vi "Combine Vectors.vi"(10 "Rotation Module Data":T1 {"Angle" scale format="%.3f"; "Velocity" scale=-1.0..1.0 scale format="%.1f"}, 11 "Travers Module Data":T1 {"Angle" scale format="%.3f"; "Velocity" scale=-1.0..1.0 scale format="%.1f"}) -> (2 "Velocity Out":dbl, 3 "Combine Out":T1 {"Angle" scale format="%.3f"; "Velocity" scale=-1.0..1.0 scale format="%.1f"})   [LabVIEW 2023, in "SwerveDrive_ACT.lvlib"]
uses:
  SwerveDrive_ACT.lvlib
  Shared Code/TypeDefs/Cluster_Module Velocity-Direction-Rotations.ctl
  Shared Code/TypeDefs/Level_Velocity plus-minus 1.ctl
  Shared Code/TypeDefs/Dial_Compase heading unit circle CCW positive.ctl
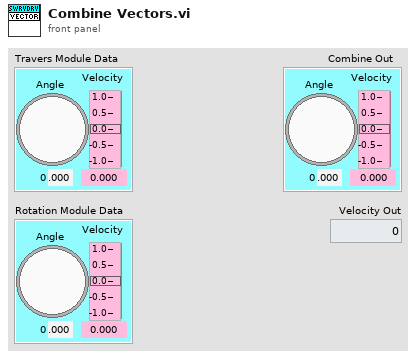
[diagram p1: front panel]
types:
  T1 = typedef "Cluster_Module Velocity-Direction-Rotations.ctl" = cluster{"Velocity":T2, "Angle":T3, "Rotations Count":dbl}
  T2 = typedef "Level_Velocity plus-minus 1.ctl" = dbl
  T3 = typedef "Dial_Compase heading unit circle CCW positive.ctl" = dbl
  T4 = typedef "Cluster_X-Y.ctl" = cluster{"X":dbl, "Y":dbl}
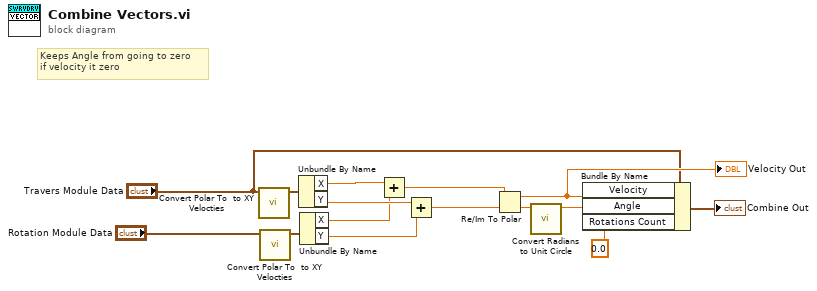
[diagram p0: block diagram]
diagram:
  # "Keeps Angle from going to zero\nif velocity it zero"
  n1 = call "Convert Polar To  to XY Velocties.vi"("Traverse"="Travers Module Data") -> ("XY Velocities Out"=w7:T4)  [unwired: 10 in]
  n2 = call "Convert Polar To  to XY Velocties.vi"("Traverse"="Rotation Module Data") -> ("XY Velocities Out"=w6:T4)  [unwired: 10 in]
  n3 = Unbundle By Name(w7) -> ("X"=w11:dbl, "Y"=w10:dbl)
  n4 = Unbundle By Name(w6) -> ("X"=w9:dbl, "Y"=w8:dbl)
  n5 = Add(x=w11, y=w9) -> (x+y=w3:dbl)
  n6 = Add(x=w10, y=w8) -> (x+y=w4:dbl)
  n7 = Re/Im To Polar(2:w4, 3:w3) -> (0:w15:dbl, 1:w12:dbl)
  "Velocity Out" <- w12
  n8 = call "Convert Radians to Unit Circle.vi"("Radians"=w15) -> ("Unit Circle"=w14:dbl)  [unwired: 10 in]
  n9 = Bundle By Name(cluster="Travers Module Data", "Velocity"=w12, "Angle"=w14, "Rotations Count"=0.0 ("Rotations")) -> (→"Combine Out":T1)
